vi "Send SCPI command.vi"(7 "Send SCPI Command":string="*TRG;", 8 "error in (no error)":errorcluster, 11 "VISA resource name":refnum<visa-resource-name>) -> (0 "error out":errorcluster, 3 "VISA resource name out":refnum<visa-resource-name>)   [LabVIEW 2015]
doc: "A low-level VI that sends a SCPI (Instrument Native Commands) to the instrument.\n\n<B>Note:</B> \n\nUse this VI only with other low-level VIs. The high-level VIs automatically incorporate this functionality. \n\nThis VI does not check the instrument status. Typically, you call this VI only in a sequence of calls to other low-level instrument driver VIs. The sequence performs one operation. You use the low-level VIs to optimize one or more aspects of interaction with the instrument. If you want to check the instrument status, call the Error Query VI at the conclusion of the sequence."
panel:
  out "token string":string
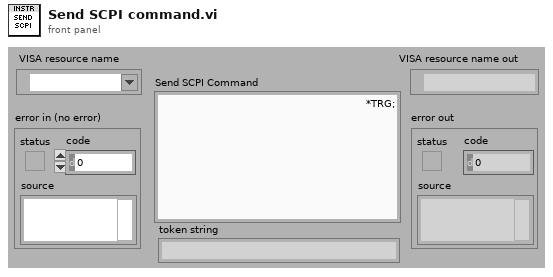
[diagram p1: front panel]
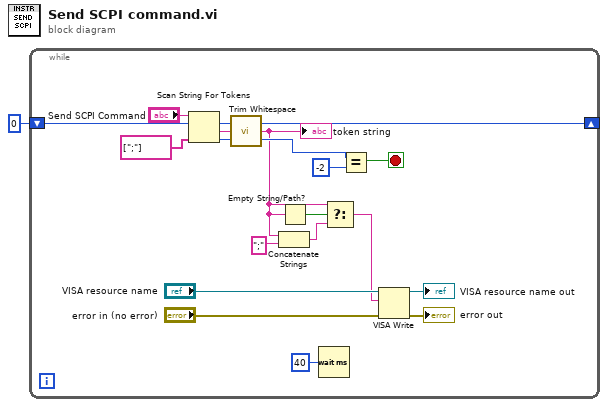
[diagram p0: block diagram]
diagram:
  n1 = while {
    shift-right: [w7] -> _
    shift-left: 0 ("token index") -> [w9]
    stop <- w12 stop-if-true
    n2 = Scan String For Tokens(6:string[] [";"] ("delimiters (\\s,\\t,\\r,\\n)"), 8:w9, 9:"Send SCPI Command") -> (0:w8:i32, 1:w13:string, 2:w7:i32)  [unwired: 3 in, 1 out]
    n3 = call <vilib>:"Trim Whitespace.vi"("string"=w13) -> ("trimmed string"=w2:string)  [unwired: 1 in]
    "token string" <- w2
    n4 = Concatenate Strings(w2, ";") -> (w4:string)
    n5 = Empty String/Path?(string/path=w2) -> (empty?=w5:bool)
    n6 = Wait (ms)(milliseconds to wait=u32 40) -> ()  [unwired: 1 out]
    n7 = Select(t=w2, s=w5, f=w4) -> (s? t:f=w3:string)
    n8 = Equal?(x=w8, y=-2) -> (x = y?=w12:bool)
    n9 = VISA Write(VISA resource name="VISA resource name", write buffer=w3, error in (no error)="error in (no error)") -> (VISA resource name out=→"VISA resource name out":refnum<visa-resource-name>, error out=→"error out":errorcluster)  [unwired: 1 out]
  }
